vi "Voltage_Divider.vi"() -> ()   [LabVIEW 2022 SP3]
panel:
  in  "R1":sgl=3.0 step=0.2
  in  "R2":sgl=2.0 step=0.2
  out "Voltage at R2":dbl
  in  "Vs Control":sgl(knob) scale=0.0..12.0
  # "R1"
  # "Voltage_Divider:\nFor the given circuit to the right,\nselect values for both R1 and R2.\nThen choose a Voltage for the power\nsupply to find the voltage across R2."
  # "R2"
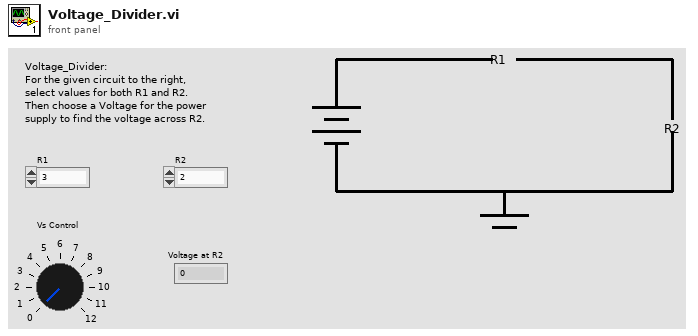
[diagram p1: front panel]
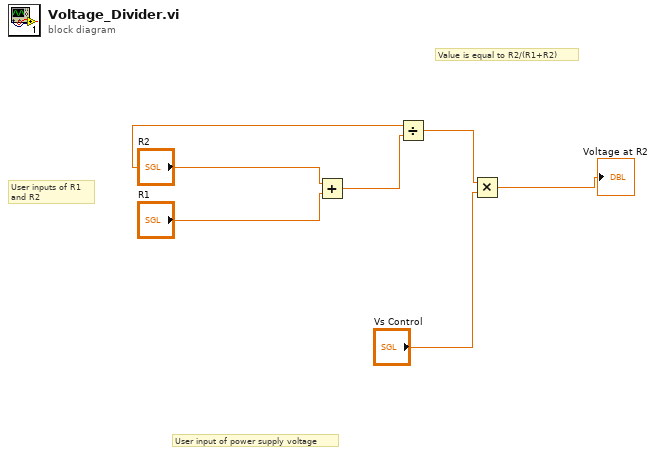
[diagram p0: block diagram]
diagram:
  # "User input of power supply voltage"
  # "Value is equal to R2/(R1+R2)"
  # "User inputs of R1\nand R2"
  n1 = Add(x="R2", y="R1") -> (x+y=w4:sgl)
  n2 = Divide(x="R2", y=w4) -> (x/y=w3:sgl)
  n3 = Multiply(x=w3, y="Vs Control") -> (x*y=→"Voltage at R2":sgl)
